vi "Handle Stat Sections.vi"(0 "StatBundle In":T1(array[cluster]), 5 "CMD Step":dbl format="%#_13g", 7 "DesiredParameters":T2, 9 "LastDataSet":string[](array[string]), 11 "Controller?":bool) -> (4 "StatBundle Out":T1(array[cluster]))   [LabVIEW 2019]
uses:
  TypeDef/Command Cluster.ctl
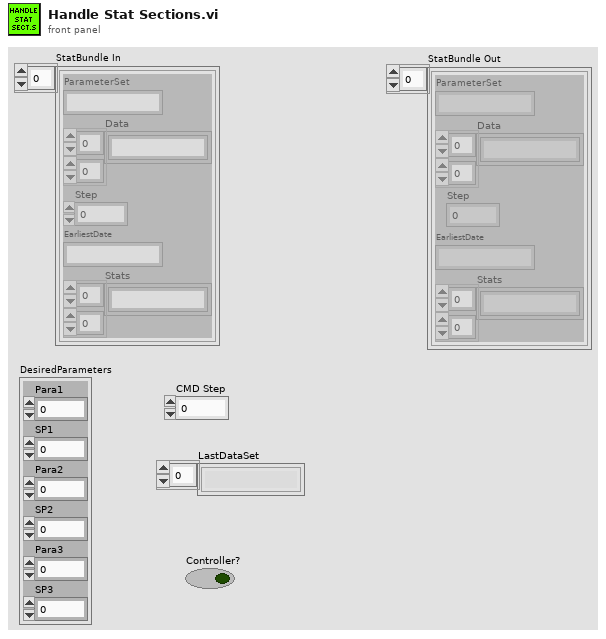
[diagram p1: front panel]
types:
  T1 = cluster{"ParameterSet":string, "Data":string[][], "Step":i32, "EarliestDate":string, "Stats":string[][]}[]
  T2 = typedef "Command Cluster.ctl" = cluster{"Para1":i32, "SP1":dbl, "Para2":i32, "SP2":dbl, "Para3":i32, "SP3":dbl}
  T3 = cluster{"ParameterSet":string, "Data":string[][], "Step":i32, "EarliestDate":string, "Stats":string[][]}
  T4 = cluster{"EarliestDate":string, cluster{"ParameterSet":string, "Data":string[][], "Step":i32, "EarliestDate":string, "Stats":string[][]}}
  T5 = cluster{"EarliestDate":string, cluster{"ParameterSet":string, "Data":string[][], "Step":i32, "EarliestDate":string, "Stats":string[][]}}[]
  T6 = cluster{"Step":i32, cluster{"ParameterSet":string, "Data":string[][], "Step":i32, "EarliestDate":string, "Stats":string[][]}}
  T7 = cluster{"Step":i32, cluster{"ParameterSet":string, "Data":string[][], "Step":i32, "EarliestDate":string, "Stats":string[][]}}[]
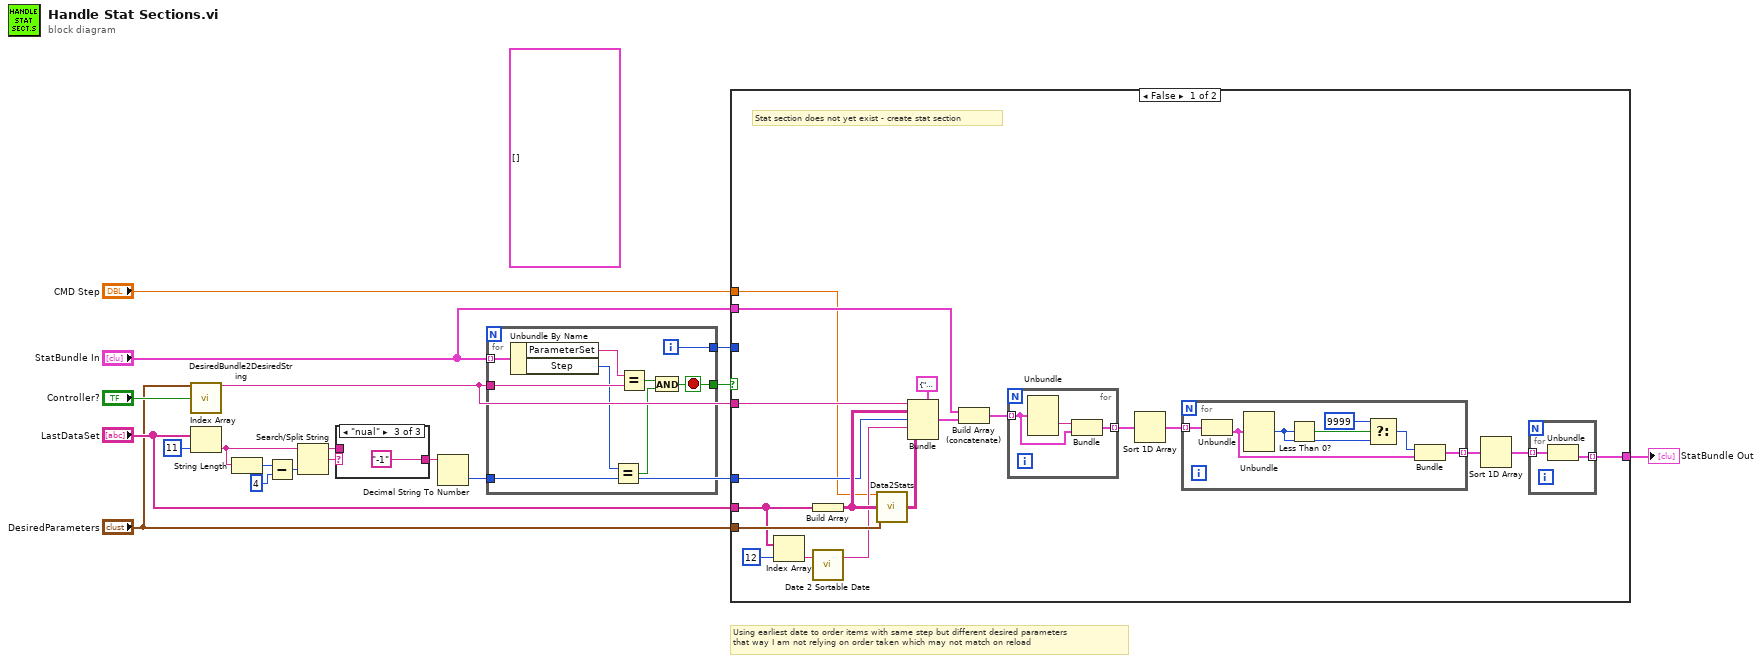
[diagram p0: block diagram]
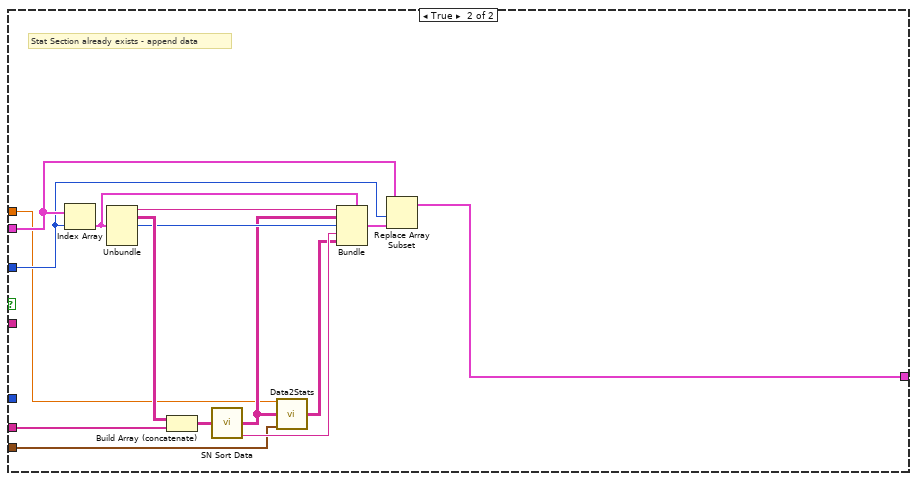
[diagram p2: hidden frame]
diagram:
  (unwired) T1 []
  # "Using earliest date to order items with same step but different desired parameters\nthat way I am not relying on order taken which may not match on reload"
  n1 = call "DesiredBundle2DesiredString.vi"("DesiredParameters"="DesiredParameters", "Controller?"="Controller?") -> ("ParameterSet"=w2:string)  [unwired: 13 in]
  n2 = Index Array(array="LastDataSet", index=11) -> (element=w18:string)
  n3 = String Length(string=w18) -> (length=w11:i32)
  n4 = Subtract(x=w11, y=4) -> (x-y=w14:i32)
  n5 = Search/Split String(string=w18, offset (0)=w14) -> (substring before match=w15:string, match + rest of string=w13:string)  [unwired: 1 in, 1 out]
  n6 = case shown="\"nual\"" w13 {
    selector: w13 -> [w19 _ _]
    tunnel: [w19 w20 "-1"] -> w16
    tunnel: w15 -> [_ w20 _]
    frame Default {
    }
    frame " (M)" {
    }
    frame "nual" {
    }
  }
  n7 = Decimal String To Number(string=w16) -> (number=w7:i32)  [unwired: 2 in, 1 out]
  n8 = for {
    tunnel: "StatBundle In" -> [w30] mode=indexing
    tunnel: w7 -> [w27]
    tunnel: w2 -> [w29]
    tunnel: [w23] -> w9
    tunnel: [w22] -> w10
    i -> [w23]
    stop <- w22 stop-if-true
    n9 = Unbundle By Name(w30) -> ("ParameterSet"=w28:string, "Step"=w26:i32)
    n10 = Equal?(x=w26, y=w27) -> (x = y?=w24:bool)
    n11 = Equal?(x=w28, y=w29) -> (x = y?=w25:bool)
    n12 = And(x=w25, y=w24) -> (x .and. y?=w22:bool)
  }
  n13 = case shown="False" w10 {
    tunnel: w9 -> [_ w73]
    tunnel: "StatBundle In" -> [w40 w76]
    tunnel: "LastDataSet" -> [w46 w70]
    tunnel: "DesiredParameters" -> [w47 w64]
    tunnel: w2 -> [w42 _]
    tunnel: w7 -> [w41 _]
    tunnel: [w32 w63] -> w6
    tunnel: "CMD Step" -> [w31 w62]
    frame False {
      # "Stat section does not yet exist - create stat section"
      n14 = Index Array(array=w46, index=12) -> (element=w44:string)
      n15 = Build Array(w46) -> (w48:string[][])
      n16 = call "Date 2 Sortable Date.vi"("Date String"=w44) -> ("Sortable Date"=w43:string)  [unwired: 2 in]
      n17 = call "Data2Stats.vi"("CMD Step"=w31, "DataIn"=w48, "DesiredParameters"=w47) -> ("StatsOut"=w34:string[][])  [unwired: 12 in]
      n18 = Bundle(cluster=T3 {"ParameterSet"="", "Data"=[], "Step"=0, "EarliestDate"="", "Stats"=[]}, "ParameterSet"=w42, "Data"=w48, "Step"=w41, "EarliestDate"=w43, "Stats"=w34) -> (w39:T3)
      n19 = Build Array (concatenate)(w40, w39) -> (w38:T1)
      n20 = for {
        tunnel: w38 -> [w61] mode=indexing
        tunnel: [w59] -> w37 mode=indexing
        n21 = Unbundle(w61) -> ("EarliestDate"=w60:string)  [unwired: 4 out]
        n22 = Bundle("EarliestDate"=w60, w61) -> (w59:T4)  [unwired: 1 in]
      }
      n23 = Sort 1D Array(array=w37) -> (sorted array=w36:T5)
      n24 = for {
        tunnel: w36 -> [w58] mode=indexing
        tunnel: [w57] -> w35 mode=indexing
        n25 = Unbundle(w58) -> (w56:T3)  [unwired: 1 out]
        n26 = Unbundle(w56) -> ("Step"=w54:i32)  [unwired: 4 out]
        n27 = Less Than 0?(x=w54) -> (x < 0?=w55:bool)
        n28 = Select(t=9999, s=w55, f=w54) -> (s? t:f=w52:i32)
        n29 = Bundle("Step"=w52, w56) -> (w57:T6)  [unwired: 1 in]
      }
      n30 = Sort 1D Array(array=w35) -> (sorted array=w33:T7)
      n31 = for {
        tunnel: w33 -> [w51] mode=indexing
        tunnel: [w50] -> w32 mode=indexing
        n32 = Unbundle(w51) -> (w50:T3)  [unwired: 1 out]
      }
    }
    frame True {
      # "Stat Section already exists - append data"
      n33 = Index Array(array=w76, index=w73) -> (element=w75:T3)
      n34 = Unbundle(w75) -> ("ParameterSet"=w72:string, "Data"=w71:string[][], "Step"=w67:i32)  [unwired: 2 out]
      n35 = Build Array (concatenate)(w71, w70) -> (w69:string[][])
      n36 = call "SN Sort Data.vi"("Array In"=w69) -> ("Array Out"=w66:string[][], "EarliestDate"=w68:string)  [unwired: 13 in]
      n37 = call "Data2Stats.vi"("CMD Step"=w62, "DataIn"=w66, "DesiredParameters"=w64) -> ("StatsOut"=w65:string[][])  [unwired: 12 in]
      n38 = Bundle(cluster=w75, "ParameterSet"=w72, "Data"=w66, "Step"=w67, "EarliestDate"=w68, "Stats"=w65) -> (w74:T3)
      n39 = Replace Array Subset(array=w76, new element=w74, index=w73) -> (w63:T1)
    }
  }
  "StatBundle Out" <- w6
